vi "Dispense on baseplate v3.vi"   [LabVIEW 2016]
uses:
  Classes/Workspace/Fixture Enum.ctl
  Classes/Routine/Routine Enum.ctl
  Classes/Workspace/Fixture.lvclass
  Classes/Routine/Routine.lvclass
  Classes/Controller/Controller.lvclass
types:
  T1 = typedef "Routine.lvclass/Routine Enum.ctl" = enum16{"Primary Pick Up", "Pick Up All", "Put Down Secondary", "Put Down All", "Release Syringe", "Secondary Pick Up", "Secure Syringe", "Dispense on Plate", "Dispense on Kapton", "Dispense on Sensor"}
  T2 = typedef "Fixture.lvclass/Fixture Enum.ctl" = enum16{"Assembly Tray", "Syringe Space", "Component", "Pick Up Tool", "Current Position"}
  T3 = typedef "Controller.lvclass/Controllers.ctl" = cluster{"I-O.lvclass":refnum<class "I-O.lvclass">, "Motion.lvclass":refnum<class "Motion.lvclass">, "Dispenser.lvclass":refnum<class "Dispenser.lvclass">}
  T4 = typedef "Fixture.lvclass/Workspace.ctl" = cluster{"XYZTheta":dbl[], "Workspace Valve":i32, "Workspace Sensor":i32}
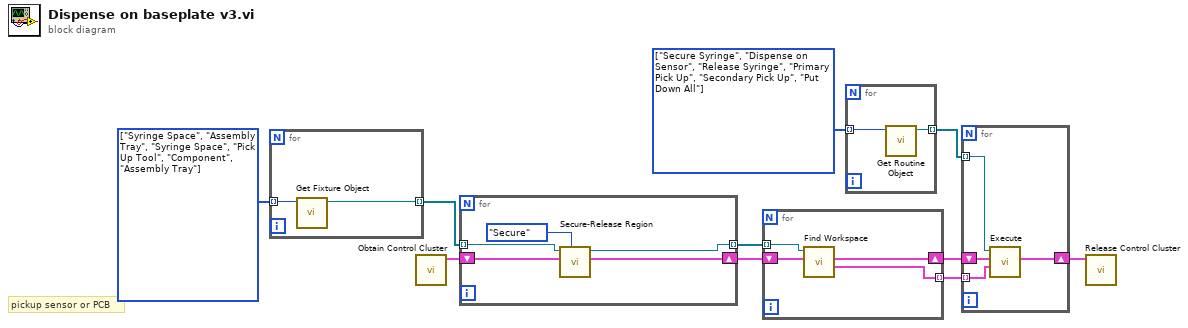
[diagram p0: block diagram]
diagram:
  w2 = T1[] [enum."Secure Syringe", enum."Dispense on Sensor", enum."Release Syringe", enum."Primary Pick Up", enum."Secondary Pick Up", enum."Put Down All"] items=["Primary Pick Up", "Pick Up All", "Put Down Secondary", "Put Down All", "Release Syringe", "Secondary Pick Up", "Secure Syringe", "Dispense on Plate", "Dispense on Kapton", "Dispense on Sensor"]
  w4 = T2[] [enum."Syringe Space", enum."Assembly Tray", enum."Syringe Space", enum."Pick Up Tool", enum."Component", enum."Assembly Tray"] items=["Assembly Tray", "Syringe Space", "Component", "Pick Up Tool", "Current Position"]
  # "pickup sensor or PCB"
  n1 = for {
    tunnel: w4 -> [w12] mode=indexing
    tunnel: [w11] -> w3 mode=indexing
    n2 = call "Get Fixture Object.vi"("Fixture"=w12) -> ("Fixture.lvclass"=w11:refnum<class "Fixture.lvclass">)  [unwired: 8 in, 2 out]
  }
  n3 = call "Obtain Control Cluster.vi"() -> ("Control Out"=w9:T3)  [unwired: 11 in]
  n4 = for {
    tunnel: w3 -> [w17] mode=indexing
    tunnel: [w16] -> w10 mode=indexing
    shift-right: [w14] -> w8
    shift-left: w9 -> [w15]
    n5 = call-dynamic "Secure-Release Region.vi"("Action"=enum16{"Secure", "Release"}."Secure", "Control In"=w15, "Fixture in"=w17) -> ("Control Out"=w14:T3, "Fixture out"=w16:refnum<class "Fixture.lvclass">)  [unwired: 6 in, 1 out]
  }
  n6 = for {
    tunnel: w10 -> [w21] mode=indexing
    shift-right: [w19] -> w7
    shift-left: w8 -> [w20]
    tunnel: [w18] -> w5 mode=indexing
    n7 = call-dynamic "Find Workspace.vi"("Control In"=w20, "Workspace In"=w21) -> ("Workspace Out"=w18:T4, "Control Out"=w19:T3)  [unwired: 6 in, 2 out]
  }
  n8 = for {
    tunnel: w2 -> [w23] mode=indexing
    tunnel: [w22] -> w1 mode=indexing
    n9 = call "Get Routine Object.vi"("Routine"=w23) -> ("Routine out"=w22:refnum<class "Routine.lvclass">)  [unwired: 9 in, 1 out]
  }
  n10 = for {
    shift-right: [w26] -> w6
    shift-left: w7 -> [w27]
    tunnel: w5 -> [w25] mode=indexing
    tunnel: w1 -> [w24] mode=indexing
    n11 = call-dynamic "Execute.vi"("Workspace"=w25, "Control In"=w27, "Routine in"=w24) -> ("Control Out"=w26:T3)  [unwired: 6 in, 2 out]
  }
  n12 = call "Release Control Cluster.vi"("output cluster"=w6) -> ()  [unwired: 11 in]
